vi "Update Template Graph.vi"(6 "Set Task Info?":bool, 8 "error in (no error)":errorcluster, 9 "Update Axes Scale":bool, 10 "Task Info In":T1={"Number of Trials"=1, "Sampling Rate (Hz)"=200, "Trial Duration (s)"=10, "Adjusted MVC (N)"=5.0, "R Phase"=0, "L Phase"=0, "L Pattern"=1, "R Pattern"=1, "Time Between Trials (s)"=5, "Lissajous Speed"=200} {"Lissajous Speed" min=1 max=200; "Time Between Trials (s)" min=1 step=1; "R Pattern" min=1 max=20 step=1; "L Pattern" min=1 max=20 step=1; "L Phase" max=360 step=1; "R Phase" max=360 step=1; "Adjusted MVC (N)" min=1.0 step=1.0; "Trial Duration (s)" min=1 step=1; "Sampling Rate (Hz)" min=1 step=1; "Number of Trials" min=1 step=1}, 11 "NI Force Task in":refnum<class "NI Force Task.lvclass">) -> (0 "error out":errorcluster, 3 "NI Force Task out":refnum<class "NI Force Task.lvclass">)   [LabVIEW 2020, in "NI Force Task.lvlib" / "NI Force Task.lvclass"]
uses:
  NI Force Task.lvclass
  Task info df.ctl
  NI Force Task.lvclass/NI Force Task.ctl
  <vilib>/Utility/miscctls.llb/LVBoundsTypeDef.ctl
  <vilib>/Analysis/1siggen.llb/Ramp Pattern by Samples.vi
  <vilib>/express/express arith-compare/Formula/XNode/ExpressFormulaBlockNode.xnode
  <vilib>/ActorFramework/Message Enqueuer/Message Enqueuer.lvclass
  <vilib>/Analysis/NI_AALBase.lvlib
  Lissajous Viewer Messages/Update graph Msg/Update graph Msg.lvclass
panel:
  # "Left Arm"
  # "Right Arm"
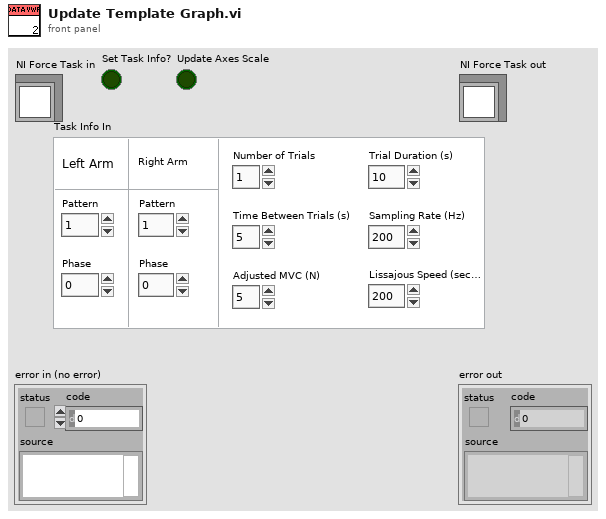
[diagram p1: front panel]
types:
  T1 = typedef "Task info df.ctl" = cluster{"Number of Trials":u8, "Sampling Rate (Hz)":u16, "Trial Duration (s)":u8, "Adjusted MVC (N)":dbl, "R Phase":i32, "L Phase":i32, "L Pattern":u8, "R Pattern":u8, "Time Between Trials (s)":u8, "Lissajous Speed":u16}
  T2 = typedef "LVBoundsTypeDef.ctl" = cluster{"Width":u32, "Height":u32}
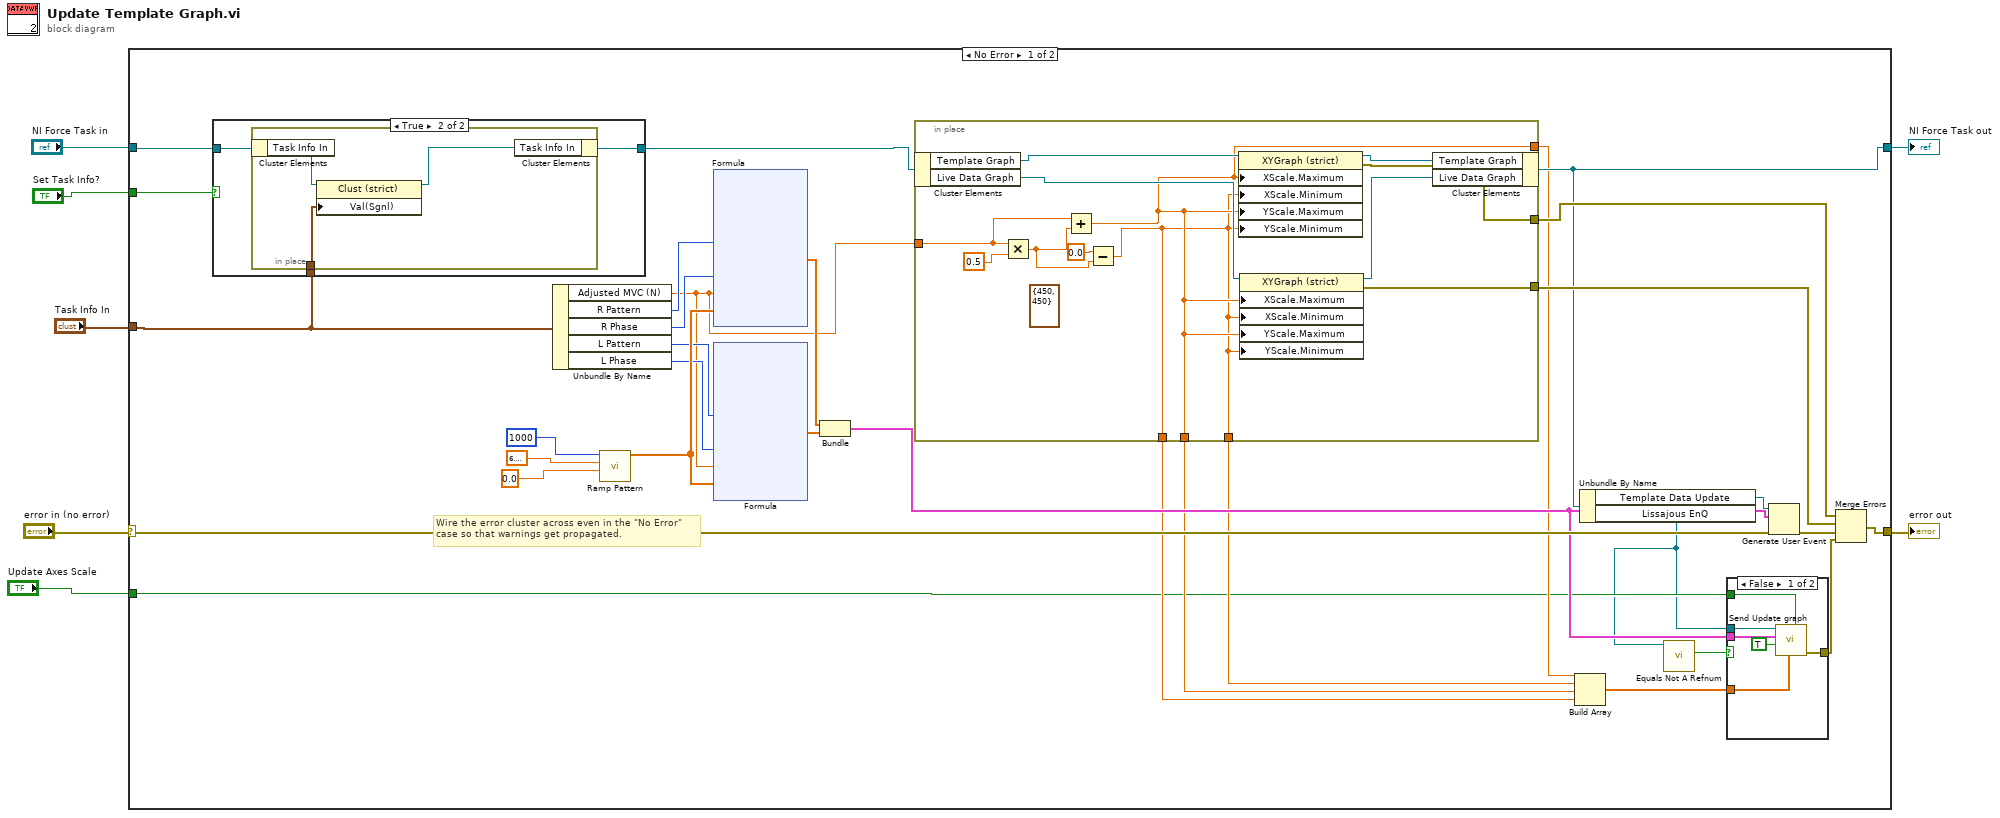
[diagram p0: block diagram]
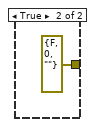
[diagram p2: hidden frame]
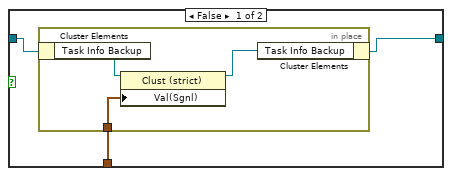
[diagram p3: hidden frame]
diagram:
  n1 = case shown="No Error" "error in (no error)" {
    selector: "error in (no error)" -> [w29 w110]
    tunnel: [w26 w110] -> w6
    tunnel: [w22 w109] -> w4
    tunnel: "NI Force Task in" -> [w21 w109]
    tunnel: "Task Info In" -> [w20 _]
    tunnel: "Set Task Info?" -> [w11 _]
    tunnel: "Update Axes Scale" -> [w10 _]
    frame No Error {
      # "Wire the error cluster across even in the \"No Error\"\ncase so that warnings get propagated."
      n2 = case shown="True" w11 {
        tunnel: w21 -> [w61 w67]
        tunnel: w20 -> [w60 w66]
        tunnel: [w59 w65] -> w19
        frame False {
          n3 = in-place {
            in-place-border: w60 -> [w63]
            n4 = in-place-cluster #1(w61) -> ("Task Info Backup"=w64:refnum<vi>)
            n5 = property class="Clust (strict)"(reference=w64, "Val(Sgnl)"=w63) -> (reference out=w62:refnum<vi>)  [unwired: 1 in, 1 out]
            n6 = in-place-cluster #1("Task Info Backup"=w62) -> (w59:refnum<class "NI Force Task.lvclass">)
          }
        }
        frame True {
          n7 = in-place {
            in-place-border: w66 -> [w68]
            n8 = in-place-cluster #2(w67) -> ("Task Info In"=w70:refnum<vi>)
            n9 = property class="Clust (strict)"(reference=w70, "Val(Sgnl)"=w68) -> (reference out=w69:refnum<vi>)  [unwired: 1 in, 1 out]
            n10 = in-place-cluster #2("Task Info In"=w69) -> (w65:refnum<class "NI Force Task.lvclass">)
          }
        }
      }
      n11 = Unbundle By Name(w20) -> ("Adjusted MVC (N)"=w28:dbl, "R Pattern"=w35:u8, "R Phase"=w34:i32, "L Pattern"=w33:u8, "L Phase"=w32:i32)
      n12 = call-poly <vilib>:"Ramp Pattern.vi"("start"=0.0, "end"=6.283185307179586, "samples"=1000) -> ("Ramp Pattern"=w36:dbl[])  [unwired: 7 in, 1 out]
      n13 = xnode "Formula"("kx"=w35, "p"=w34, "nR"=w28, "t"=w36) -> ("Result"=w31:dbl[])  [unwired: 1 in, 1 out]
      n14 = xnode "Formula"("ky"=w33, "c"=w32, "nR"=w28, "t"=w36) -> ("Result"=w30:dbl[])  [unwired: 1 in, 1 out]
      n15 = Bundle("Result"=w31, "Result"=w30) -> (w18:cluster{"Result":dbl[], "Result":dbl[]})  [unwired: 1 in]
      n16 = in-place {
        in-place-border: w28 -> [w53]
        in-place-border: [w56] -> w25
        in-place-border: [w55] -> w24
        in-place-border: [w48] -> w16
        in-place-border: [w47] -> w15
        in-place-border: [w48] -> w14
        in-place-border: [w47] -> w13
        (unwired) T2 {"Width"=450, "Height"=450} ("Plot Area:Size")
        n17 = in-place-cluster #3(w19) -> ("Template Graph"=w50:refnum<vi>, "Live Data Graph"=w49:refnum<vi>)
        n18 = Multiply(x=w53, y=sgl 0.5 ("Adjusted MVC (N)")) -> (x*y=w51:dbl)
        n19 = Add(x=w53, y=w51) -> (x+y=w48:dbl)
        n20 = Subtract(x=0.0, y=w51) -> (x-y=w47:dbl)
        n21 = property class="XYGraph (strict)"(reference=w50, "XScale.Maximum"=w48, "XScale.Minimum"=w47, "YScale.Maximum"=w48, "YScale.Minimum"=w47) -> (reference out=w58:refnum<vi>, error out=w55:errorcluster)  [unwired: 1 in]
        n22 = property class="XYGraph (strict)"(reference=w49, "XScale.Maximum"=w48, "XScale.Minimum"=w47, "YScale.Maximum"=w48, "YScale.Minimum"=w47) -> (reference out=w57:refnum<vi>, error out=w56:errorcluster)  [unwired: 1 in]
        n23 = in-place-cluster #3("Template Graph"=w58, "Live Data Graph"=w57) -> (w22:refnum<class "NI Force Task.lvclass">)
      }
      n24 = Build Array(w16, w15, w14, w13) -> (w12:dbl[])
      n25 = Unbundle By Name(w22) -> ("Template Data Update"=w23:refnum<user-event>, "Lissajous EnQ"=w9:refnum<class "Message Enqueuer.lvclass">)
      n26 = call <vilib>:"Equals Not A Refnum.vi"("Message Enqueuer"=w9) -> ("Not a refnum?"=w8:bool)  [unwired: 10 in]
      n27 = case shown="False" w8 {
        tunnel: w9 -> [w45 _]
        tunnel: w18 -> [w44 _]
        tunnel: [w42 errorcluster {"status"=FALSE, "code"=0, "source"=""} ("error out")] -> w17
        tunnel: w12 -> [w41 _]
        tunnel: w10 -> [w40 _]
        frame False {
          n28 = call "Send Update graph.vi"("Set Axis Scale?"=w40, "X and Y scaling"=w41, "Template?"=TRUE, "Data"=w44, "Message Enqueuer in"=w45) -> ("error out"=w42:errorcluster)  [unwired: 5 in, 1 out]
        }
        frame True {
        }
      }
      n29 = Generate User Event(user event=w23, event data cluster=w18, error in=w29) -> (error out=w27:errorcluster)  [unwired: 1 in, 1 out]
      n30 = Merge Errors(w24, w25, w27, w17) -> (w26:errorcluster)
    }
    frame Error {
    }
  }
  "error out" <- w6
  "NI Force Task out" <- w4
